vi "datacollection.vi"(8 "stop":bool, 10 "rate":dbl=1000.0 format="%0.2f", 11 "samples per channel":i32=1000) -> (1 "error out":errorcluster, 2 "All Sensors":dynamicdata(graph), 6 "SampClk.Rate Indicator":dbl, 7 "Elapsed Time":dbl)   [LabVIEW 2022 SP3]
uses:
  <vilib>/DAQmx/read.llb/DAQmx Read (Analog 1D Wfm NChan NSamp).vi
  <vilib>/DAQmx/configure/timing.llb/DAQmx Timing (Sample Clock).vi
  <vilib>/DAQmx/miscellaneous.llb/DAQmx Fill In Error Info.vi
  <resource>/objmgr/daqmx.rc
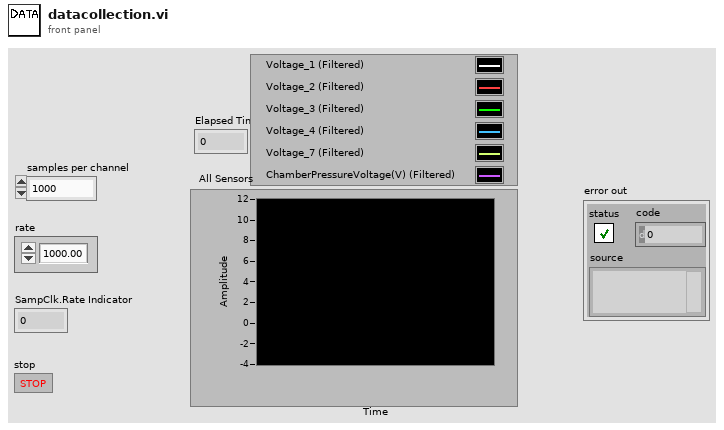
[diagram p1: front panel]
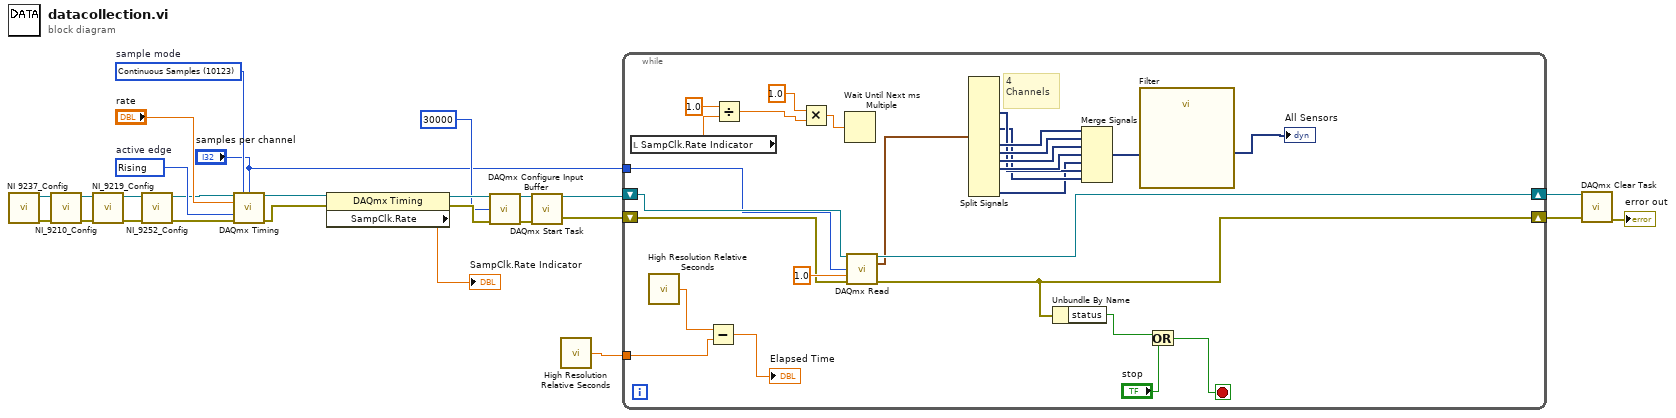
[diagram p0: block diagram]
diagram:
  w18 = 10123 items=["Finite Samples"=10178, "Continuous Samples"=10123, "Hardware Timed Single Point"=12522]  # sample mode
  w20 = 10280 items=["Rising"=10280, "Falling"=10171]  # active edge
  n1 = call "NI 9237_Config.vi"() -> ("error out"=w21:errorcluster, "task out"=w22:refnum<k21>)  [unwired: 10 in]
  n2 = call "NI_9210_Config.vi"("error in"=w21, "task in"=w22) -> ("error out"=w24:errorcluster, "task out"=w23:refnum<k21>)  [unwired: 8 in]
  n3 = call "NI_9219_Config.vi"("error in"=w24, "task in"=w23) -> ("error out"=w25:errorcluster, "task out"=w26:refnum<k21>)  [unwired: 8 in]
  n4 = call "NI_9252_Config.vi"("error in"=w25, "task in"=w26) -> ("error out"=w16:errorcluster, "task out"=w17:refnum<k21>)  [unwired: 8 in]
  n5 = call-poly <vilib>:"DAQmx Timing.vi"("task/channels in"=w17, "sample mode"=w18, "samples per channel"="samples per channel", "rate"="rate", "active edge"=w20, "error in"=w16) -> ("task out"=w15:refnum<k21>, "error out"=w14:errorcluster)  [unwired: 8 in]
  n6 = property class="DAQmx Timing"(reference=w15, error in=w14) -> (reference out=w12:refnum<k21>, error out=w11:errorcluster, "SampClk.Rate"=→"SampClk.Rate Indicator":dbl)
  n7 = call <vilib>:"DAQmx Configure Input Buffer.vi"("task/channels in"=w12, "buffer size (in samples per channel)"=u32 30000, "error in"=w11) -> ("task out"=w10:refnum<k21>, "error out"=w9:errorcluster)  [unwired: 11 in]
  n8 = call <vilib>:"DAQmx Start Task.vi"("task/channels in"=w10, "error in"=w9) -> ("task out"=w7:refnum<k21>, "error out"=w5:errorcluster)  [unwired: 12 in]
  n9 = call <vilib>:"High Resolution Relative Seconds.vi"() -> ("relative seconds"=w4:dbl)
  n10 = while {
    shift-right: [w45] -> w3
    shift-left: w7 -> [w47]
    shift-right: [w38] -> w2
    shift-left: w5 -> [w46]
    tunnel: "samples per channel" -> [w43]
    tunnel: w4 -> [w30]
    stop <- w32 stop-if-true
    # "4\nChannels"
    n11 = local read "SampClk.Rate Indicator"() -> (w49:dbl)
    n12 = call <vilib>:"High Resolution Relative Seconds.vi"() -> ("relative seconds"=w31:dbl)
    n13 = Subtract(x=w31, y=w30) -> (x-y=→"Elapsed Time":dbl)
    n14 = Divide(x=1.0, y=w49) -> (x/y=w52:dbl)
    n15 = Multiply(x=1.0, y=w52) -> (x*y=w51:dbl)
    n16 = Wait Until Next ms Multiple(millisecond multiple=w51) -> ()  [unwired: 1 out]
    n17 = call-poly <vilib>:"DAQmx Read.vi"("task/channels in"=w47, "number of samples per channel"=w43, "timeout"=1.0, "error in"=w46) -> ("task out"=w45:refnum<k21>, "data"=w44:waveform(dbl)[], "error out"=w38:errorcluster)  [unwired: 9 in]
    n18 = Split Signals(w44) -> (w37:dynamicdata, w36:dynamicdata, w39:dynamicdata, w40:dynamicdata, w41:dynamicdata, w42:dynamicdata, w27:dynamicdata)  [unwired: 15 in, 8 out]
    n19 = Unbundle By Name(w38) -> ("status"=w33:bool)
    n20 = Merge Signals(w39, w40, w41, w42, w27, w37, w36) -> (w35:dynamicdata)
    n21 = call "Filter"("Signal"=w35) -> ("Filtered Signal"=→"All Sensors":dynamicdata)  [unwired: 9 in, 1 out]
    n22 = Or(x=w33, y="stop") -> (x .or. y?=w32:bool)
  }
  n23 = call <vilib>:"DAQmx Clear Task.vi"("task in"=w3, "error in"=w2) -> ("error out"=→"error out":errorcluster)  [unwired: 13 in]
